vi "clear.vi"(8 "error in (no error)":errorcluster, 11 "InconsistentList in":refnum<class "NI_Robotics_InconsistentList.lvclass">) -> (0 "error out":errorcluster, 3 "InconsistentList out":refnum<class "NI_Robotics_InconsistentList.lvclass">)   [LabVIEW 2017, in "NI_Robotics_InconsistentList.lvclass"]
uses:
  <vilib>/robotics/Navigation/shared/InconsistentList/NI_Robotics_InconsistentList.lvclass
  <vilib>/robotics/Navigation/shared/InconsistentList/NI_Robotics_InconsistentList.lvclass/NI_Robotics_InconsistentList.ctl
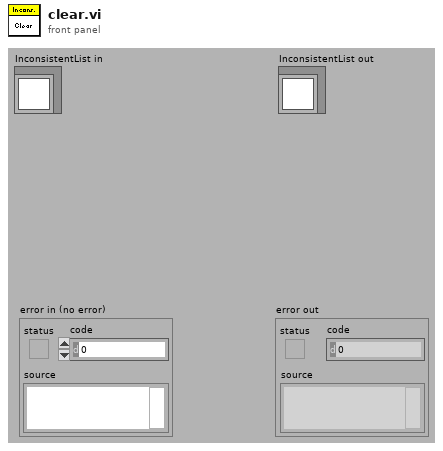
[diagram p1: front panel]
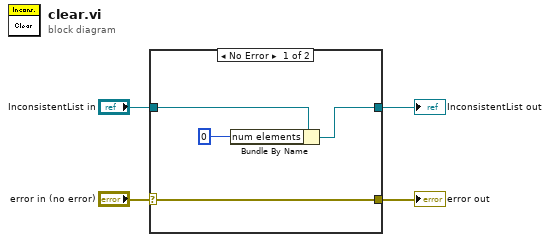
[diagram p0: block diagram]
diagram:
  n1 = case shown="No Error" "error in (no error)" {
    selector: "error in (no error)" -> [w8 w9]
    tunnel: "InconsistentList in" -> [w6 w10]
    tunnel: [w7 w10] -> w3
    tunnel: [w8 w9] -> w1
    frame No Error {
      n2 = Bundle By Name(cluster=w6, "num elements"=0) -> (w7:refnum<class "NI_Robotics_InconsistentList.lvclass">)
    }
    frame Error {
    }
  }
  "InconsistentList out" <- w3
  "error out" <- w1
